vi "Car Models.vi"(0 "body":string) -> (1 "No of HTMLs":i32, 2 "Car HTMLs":string[](array[string]))   [LabVIEW 2018]
uses:
  <vilib>/httpClient/LabVIEWHTTPClient.lvlib
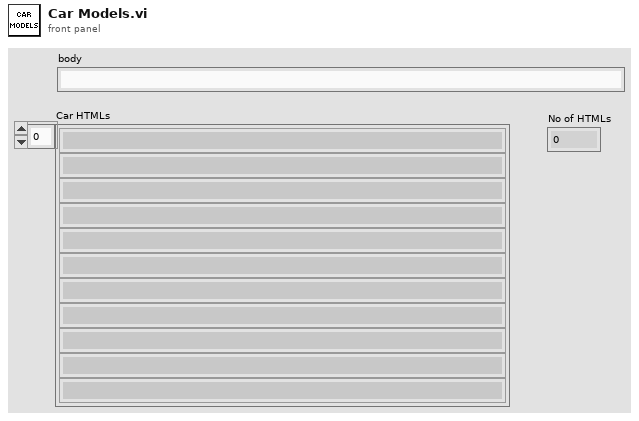
[diagram p1: front panel]
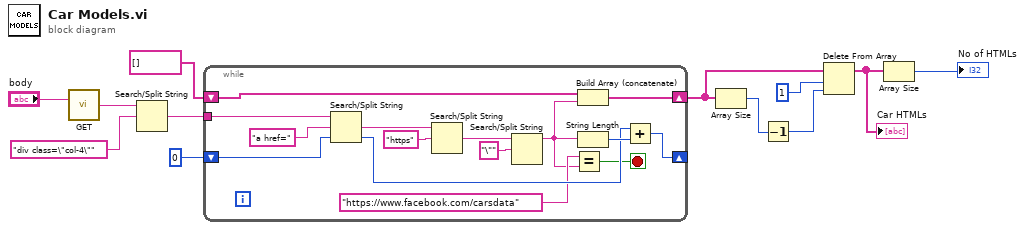
[diagram p0: block diagram]
diagram:
  n1 = call <vilib>:"GET.vi"("url"="body") -> ("body"=w8:string)  [unwired: 11 in, 3 out]
  n2 = Search/Split String(string=w8, search string/char (-)="div class=\"col-4\"") -> (match + rest of string=w12:string)  [unwired: 1 in, 2 out]
  n3 = while {
    tunnel: w12 -> [w25]
    shift-right: [w26] -> w2
    shift-left: string[] [] -> [w27]
    shift-right: [w18] -> _
    shift-left: 0 -> [w16]
    stop <- w15 stop-if-true
    n4 = Search/Split String(string=w25, search string/char (-)="a href=", offset (0)=w16) -> (match + rest of string=w20:string, offset of match=w17:i32)  [unwired: 1 out]
    n5 = Search/Split String(string=w20, search string/char (-)="https") -> (match + rest of string=w23:string)  [unwired: 1 in, 2 out]
    n6 = Search/Split String(string=w23, search string/char (-)="\"") -> (substring before match=w13:string)  [unwired: 1 in, 2 out]
    n7 = Equal?(x="https://www.facebook.com/carsdata", y=w13) -> (x = y?=w15:bool)
    n8 = Build Array (concatenate)(w27, w13) -> (w26:string[])
    n9 = String Length(string=w13) -> (length=w19:i32)
    n10 = Add(x=w17, y=w19) -> (x+y=w18:i32)
  }
  n11 = Array Size(array=w2) -> (size(s)=w4:i32)
  n12 = Decrement(x=w4) -> (x-1=w3:i32)
  n13 = Delete From Array(array=w2, length=1, index=w3) -> (array with subset deleted=w1:string[])  [unwired: 1 out]
  "Car HTMLs" <- w1
  n14 = Array Size(array=w1) -> (size(s)=→"No of HTMLs":i32)
